vi "GDSIconEditor_IconSizeAdjustment.vi"(6 "BodyIconHeightIn":i32, 7 "HideHeader":bool, 8 "ConnectorPaneHeight":i32[](array[numeric]), 9 "Frame thickness":i32, 10 "_IconSize":u16(ring) caption="Icon Size" items=["Full", "1 c-term high", "2 c-term high", "3 c-term high", "4 c-term high"], 11 "HeaderIconIn":u8[][](array[numeric]) format="%.0x") -> (1 "HeaderIconOut":u8[][](array[numeric]), 2 "BodyIconHeightOut":u32, 3 "ImageRows":i32)   [LabVIEW 2016]
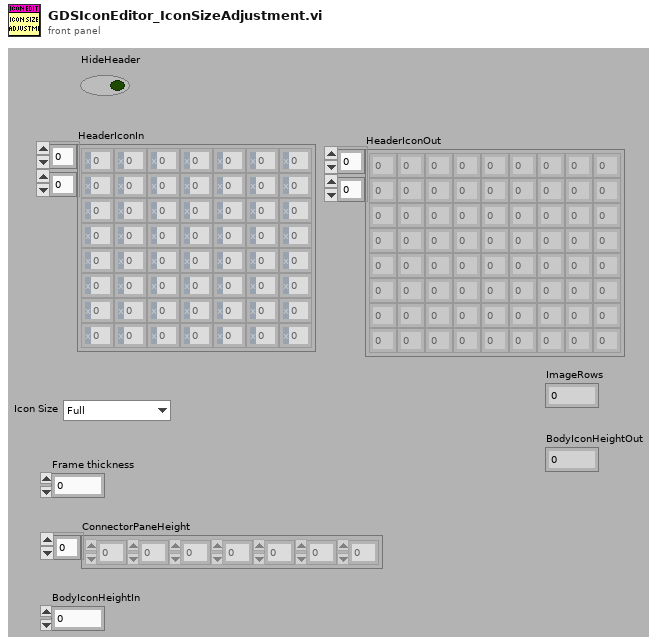
[diagram p1: front panel]
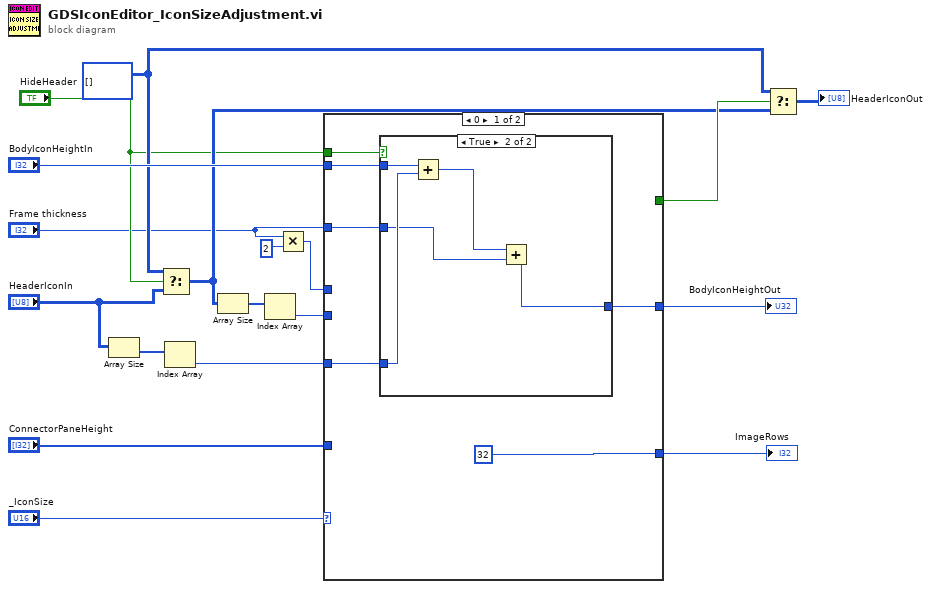
[diagram p0: block diagram]
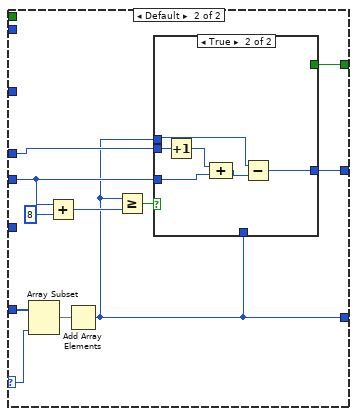
[diagram p3: hidden frame]
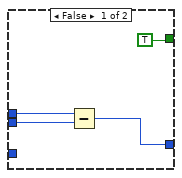
[diagram p4: hidden frame]
diagram:
  w7 = u8[][] [] ("t")
  n1 = Array Size(array="HeaderIconIn") -> (size(s)=w3:i32[])
  n2 = Select(t=w7, s="HideHeader", f="HeaderIconIn") -> (s? t:f=w6:u8[][])
  n3 = Index Array(array=w3) -> (element=w2:i32)  [unwired: 1 in]
  n4 = Array Size(array=w6) -> (size(s)=w13:i32[])
  n5 = Index Array(array=w13) -> (element=w14:i32)  [unwired: 1 in]
  n6 = Multiply(x="Frame thickness", y=u32 2) -> (x*y=w18:u32)
  n7 = case shown="0" "_IconSize" {
    selector: "_IconSize" -> [_ w38]
    tunnel: "BodyIconHeightIn" -> [w22 _]
    tunnel: [w21 w39] -> w16
    tunnel: "ConnectorPaneHeight" -> [_ w41]
    tunnel: [32 ("ImageRows(32)") w32] -> w15
    tunnel: w14 -> [_ w34]
    tunnel: w18 -> [_ w33]
    tunnel: [_ w31] -> w9
    tunnel: "HideHeader" -> [w23 _]
    tunnel: w2 -> [w20 _]
    tunnel: "Frame thickness" -> [w19 _]
    frame 0 {
      n8 = case shown="True" w23 {
        tunnel: w22 -> [w25 w30]
        tunnel: [w25 w26] -> w21
        tunnel: w20 -> [_ w29]
        tunnel: w19 -> [_ w28]
        frame False {
        }
        frame True {
          n9 = Add(x=w30, y=w29) -> (x+y=w27:i32)
          n10 = Add(x=w27, y=w28) -> (x+y=w26:i32)
        }
      }
    }
    frame Default {
      n11 = Array Subset(array=w41, length=w38) -> (w40:i32[])  [unwired: 1 in]
      n12 = Add(x=w34, y=8) -> (x+y=w36:i32)
      n13 = Add Array Elements(numeric array=w40) -> (sum=w32:i32)
      n14 = Greater Or Equal?(x=w32, y=w36) -> (x >= y?=w35:bool)
      n15 = case shown="True" w35 {
        tunnel: [w43 w51] -> w39
        tunnel: w32 -> [_ _]
        tunnel: w34 -> [_ w49]
        tunnel: w33 -> [w45 w47]
        tunnel: w32 -> [w44 w46]
        tunnel: [TRUE _] -> w31
        frame False {
          n16 = Subtract(x=w44, y=w45) -> (x-y=w43:u32)
        }
        frame True {
          n17 = Increment(x=w47) -> (x+1=w50:u32)
          n18 = Compound Arithmetic op=ADD(w50, w49) -> (w48:u32)
          n19 = Subtract(x=w46, y=w48) -> (x-y=w51:u32)
        }
      }
    }
  }
  "BodyIconHeightOut" <- w16
  "ImageRows" <- w15
  n20 = Select(t=w7, s=w9, f=w6) -> (s? t:f=→"HeaderIconOut":u8[][])
